vi "Native POST File Upload Example.vi"() -> ()   [LabVIEW 2017]
uses:
  <vilib>/httpClient/POSTFile.vi
  <vilib>/httpClient/LabVIEWHTTPClient.lvlib
panel:
  out "body":string
  out "headers":string
  in  "Authentication":cluster{"Username":string, "Password":string}
  out "error out":errorcluster
  in  "FIlepath":path=path "D:/upwork/Labview-REST-API/labview-source/payload.png"
  in  "API Endpoint Url":string="https://luferau.free.beeceptor.com/upload"
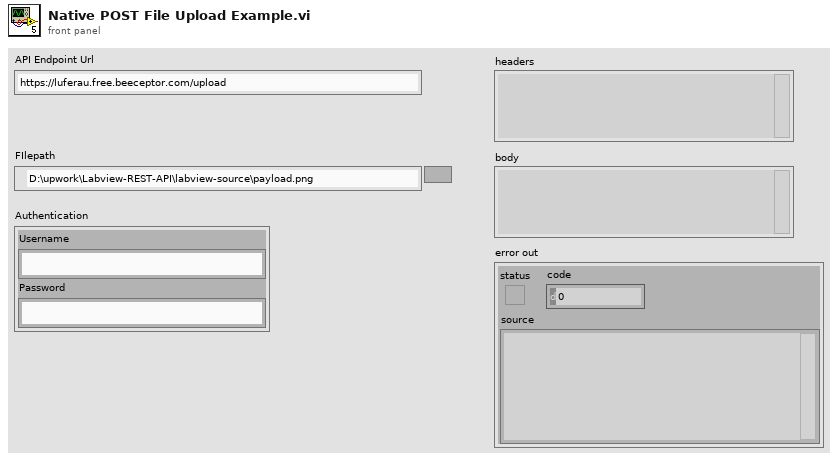
[diagram p1: front panel]
types:
  T1 = typedef "LabVIEWHTTPClient.lvlib/ClientHandle.ctl" = refnum<k1>
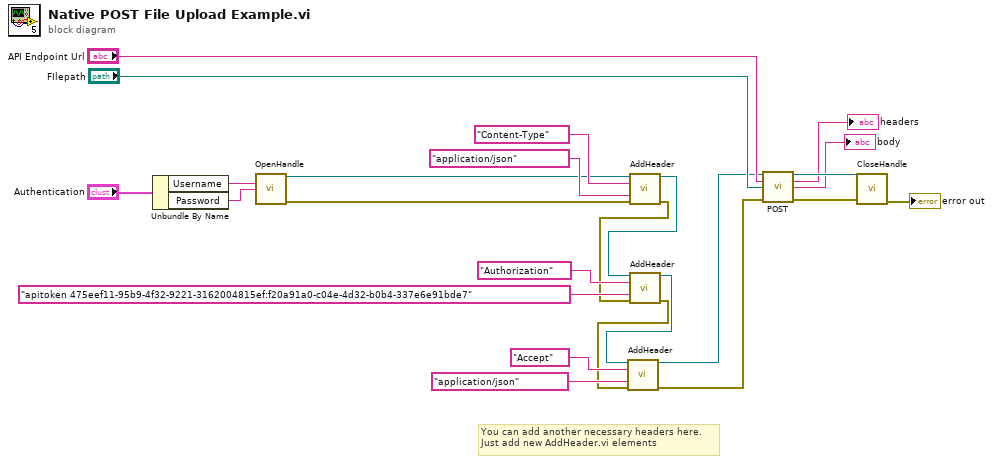
[diagram p0: block diagram]
diagram:
  # "You can add another necessary headers here.\nJust add new AddHeader.vi elements"
  n1 = Unbundle By Name("Authentication") -> ("Username"=w23:string, "Password"=w22:string)
  n2 = call <vilib>:"OpenHandle.vi"("username"=w23, "password"=w22) -> ("client handle out"=w9:T1, "error out"=w10:errorcluster)  [unwired: 12 in]
  n3 = call <vilib>:"AddHeader.vi"("client handle"=w9, "header"="Content-Type", "value"="application/json", "error in (no error)"=w10) -> ("client handle out"=w6:T1, "error out"=w5:errorcluster)  [unwired: 10 in]
  n4 = call <vilib>:"AddHeader.vi"("client handle"=w6, "header"="Authorization", "value"="apitoken 475eef11-95b9-4f32-9221-3162004815ef:f20a91a0-c04e-4d32-b0b4-337e6e91bde7", "error in (no error)"=w5) -> ("client handle out"=w4:T1, "error out"=w3:errorcluster)  [unwired: 10 in]
  n5 = call <vilib>:"AddHeader.vi"("client handle"=w4, "header"="Accept", "value"="application/json", "error in (no error)"=w3) -> ("client handle out"=w2:T1, "error out"=w1:errorcluster)  [unwired: 10 in]
  n6 = call-poly <vilib>:"POST.vi"("client handle"=w2, "url"="API Endpoint Url", "file"="FIlepath", "error in (no error)"=w1) -> ("client handle out"=w16:T1, "headers"=→"headers":string, "body"=→"body":string, "error out"=w15:errorcluster)  [unwired: 8 in]
  n7 = call <vilib>:"CloseHandle.vi"("client handle"=w16, "error in (no error)"=w15) -> ("error out"=→"error out":errorcluster)  [unwired: 13 in]
